vi "temperatureCheck.vi"() -> ()   [LabVIEW 2012]
uses:
  <vilib>/addons/database/Auxilliary.llb/DB Tools Cursor Type.ctl
  <vilib>/addons/database/Connection.llb/DB Tools Open Connec (Path).vi
  <vilib>/addons/database/Connection.llb/Conn Execute.vi
  <vilib>/addons/database/Recordset.llb/Rec Fetch Recordset Data (R).vi
  <vilib>/addons/database/Recordset.llb/Rec Destroy - Connection.vi
  <vilib>/addons/database/_DB Variant To Data/Database Variant To Data.xnode
  <vilib>/addons/database/NI_Database_API.lvlib
panel:
  out "error out 2":errorcluster
  out "concatenated string":string
  out "recordset data":variant[][](array[variant])
  out "error out":errorcluster
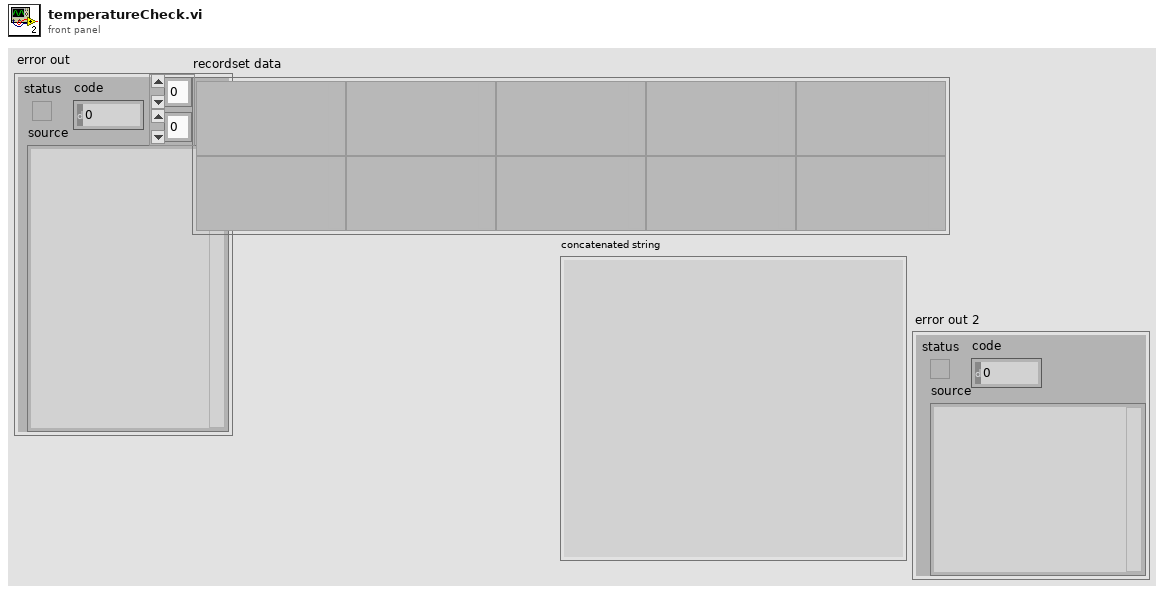
[diagram p1: front panel]
types:
  T1 = typedef "NI_Database_API.lvlib/DB Tools Cursor Type.ctl" = enum16{"forward-only", "keyset", "dynamic", "static"}
  T2 = typedef "NI_Database_API.lvlib/Conn ObjectReference.ctl" = refnum<k1>
  T3 = typedef "NI_Database_API.lvlib/Rec ObjectReference.ctl" = refnum<k1>
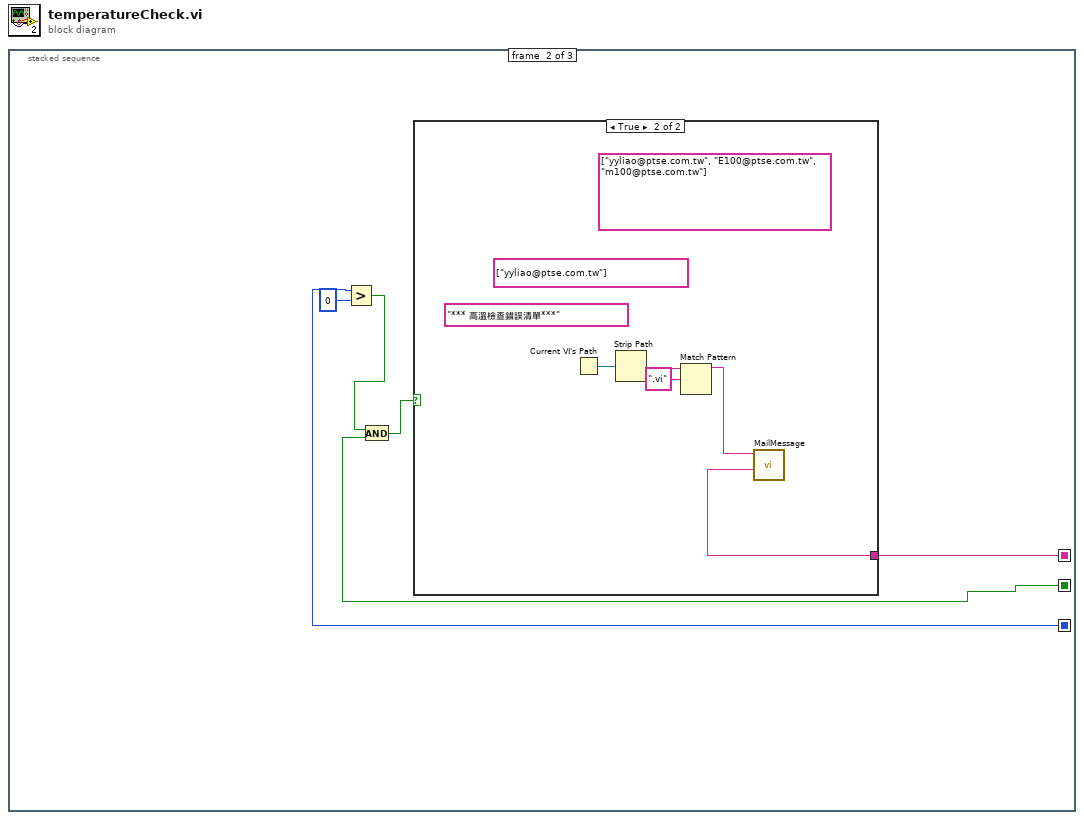
[diagram p0: block diagram]
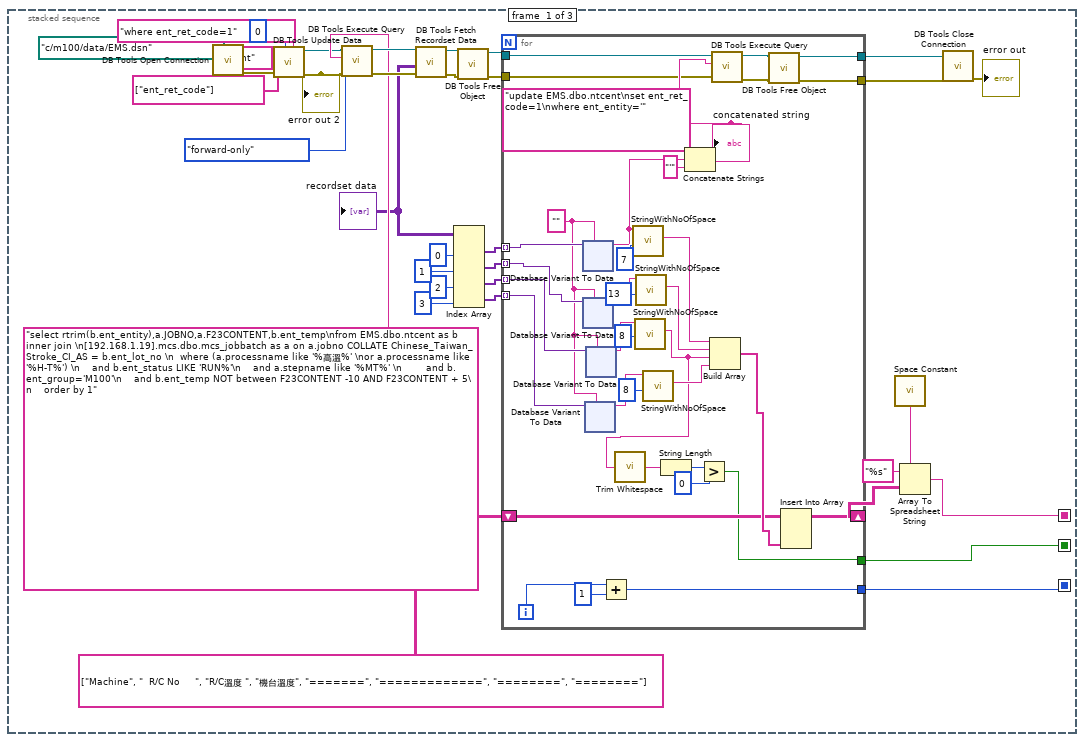
[diagram p2: hidden frame]
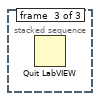
[diagram p4: hidden frame]
diagram:
  n1 = stacked-sequence {
    seq-local: [w17 _ _] -> [_ w206 _]
    seq-local: [w2 _ _] -> [_ w205 _]
    seq-local: [w1 _ _] -> [_ w201 _]
    frame #0 {
      n2 = call-poly <vilib>:"DB Tools Open Connection.vi"("connection information"=path "c:/m100/data/EMS.dsn") -> ("error out"=w8:errorcluster, "connection reference"=w10:T2)  [unwired: 7 in]
      n3 = call <vilib>:"DB Tools Update Data.vi"("condition"="where ent_ret_code=1", "data"=0, "error in (no error)"=w8, "columns"=string[] ["ent_ret_code"], "table"="ntcent", "connection reference"=w10) -> ("error out"=w7:errorcluster, "connection reference out"=w9:T2)  [unwired: 4 in]
      "error out 2" <- w7
      n4 = call-poly <vilib>:"DB Tools Execute Query.vi"("error in (no error)"=w7, "cursor type"=DB_Tools_Cursor_Type."forward-only", "SQL query"="select rtrim(b.ent_entity),a.JOBNO,a.F23CONTENT,b.ent_temp\nfrom EMS.dbo.ntcent as b inner join \n[192.168.1.19].mcs.dbo.mcs_jobbatch as a on a.jobno COLLATE Chinese_Taiwan_Stroke_CI_AS = b.ent_lot_no \n  where (a.processname like '%高溫%' \nor a.processname like '%H-T%') \n    and b.ent_status LIKE 'RUN%'\n    and a.stepname like '%MT%' \n        and b.ent_group='M100'\n    and b.ent_temp NOT between F23CONTENT -10 AND F23CONTENT + 5\n    order by 1", "connection reference"=w9) -> ("error out"=w34:errorcluster, "recordset reference"=w35:T3)  [unwired: 4 in]
      n5 = call-poly <vilib>:"DB Tools Fetch Recordset Data.vi"("error in (no error)"=w34, "recordset reference"=w35) -> ("error out"=w32:errorcluster, "recordset data"=w28:variant[][], "recordset reference out"=w33:T3)  [unwired: 3 in]
      "recordset data" <- w28
      n6 = Index Array(array=w28, index (col) #1=0 ("disabled index (col)"), index (col) #2=1 ("index (col)"), index (col) #3=2 ("index (col)"), index (col) #4=3 ("index (col)")) -> (element #1=w23:variant[], element #2=w22:variant[], element #3=w21:variant[], element #4=w20:variant[])  [unwired: 4 in]
      n7 = call-poly <vilib>:"DB Tools Free Object.vi"("error in (no error)"=w32, "recordset reference"=w33) -> ("error out"=w13:errorcluster, "connection reference"=w14:T2)  [unwired: 8 in]
      n8 = for {
        tunnel: w23 -> [w72] mode=indexing
        tunnel: w22 -> [w71] mode=indexing
        tunnel: w21 -> [w70] mode=indexing
        tunnel: w20 -> [w69] mode=indexing
        shift-right: [w66] -> w18
        shift-left: string[][] [["Machine", "  R/C No     ", "R/C溫度 ", "機台溫度"], ["=======", "=============", "========", "========"]] ("array") -> [w65]
        tunnel: w14 -> [w50]
        tunnel: w13 -> [w49]
        tunnel: [w46] -> w12
        tunnel: [w45] -> w11
        tunnel: [w42] -> w2
        tunnel: [w37] -> w1
        i -> [w44]
        w68 = ""
        n9 = xnode "Database Variant To Data"("database variant"=w72, "type"=w68) -> ("data"=w53:string)  [unwired: 1 in, 1 out]
        n10 = xnode "Database Variant To Data"("database variant"=w71, "type"=w68) -> ("data"=w57:string)  [unwired: 1 in, 1 out]
        n11 = xnode "Database Variant To Data"("database variant"=w69, "type"=w68) -> ("data"=w62:string)  [unwired: 1 in, 1 out]
        n12 = xnode "Database Variant To Data"("database variant"=w70, "type"=w68) -> ("data"=w64:string)  [unwired: 1 in, 1 out]
        n13 = Add(x=w44, y=1) -> (x+y=w42:i32)
        n14 = call "StringWithNoOfSpace.vi"("StringLength"=7, "String"=w53) -> ("OutString"=w58:string)  [unwired: 9 in]
        n15 = call "StringWithNoOfSpace.vi"("StringLength"=8, "String"=w64) -> ("OutString"=w40:string)  [unwired: 9 in]
        n16 = call <vilib>:"Trim Whitespace.vi"("string"=w40) -> ("trimmed string"=w41:string)  [unwired: 1 in]
        n17 = call "StringWithNoOfSpace.vi"("StringLength"=13, "String"=w57) -> ("OutString"=w55:string)  [unwired: 9 in]
        n18 = call "StringWithNoOfSpace.vi"("StringLength"=8, "String"=w62) -> ("OutString"=w60:string)  [unwired: 9 in]
        n19 = String Length(string=w41) -> (length=w39:i32)
        n20 = Concatenate Strings("update EMS.dbo.ntcent\nset ent_ret_code=1\nwhere ent_entity='", w53, "'" ("string")) -> (w51:string)
        "concatenated string" <- w51
        n21 = Greater?(x=w39, y=0) -> (0:w37:bool)
        n22 = Build Array(w58, w55, w40, w60) -> (w67:string[])
        n23 = call-poly <vilib>:"DB Tools Execute Query.vi"("error in (no error)"=w49, "SQL query"=w51, "connection reference"=w50) -> ("error out"=w47:errorcluster, "recordset reference"=w48:T3)  [unwired: 5 in]
        n24 = call-poly <vilib>:"DB Tools Free Object.vi"("error in (no error)"=w47, "recordset reference"=w48) -> ("error out"=w45:errorcluster, "connection reference"=w46:T2)  [unwired: 8 in]
        n25 = Insert Into Array(array=w65, new element=w67) -> (w66:string[][])  [unwired: 2 in]
      }
      n26 = call <vilib>:"Space Constant.vi"() -> ("String"=w15:string)
      n27 = Array To Spreadsheet String(delimiter (Tab)=w15, array=w18, 3:"%s" ("format string")) -> (spreadsheet string=w17:string)
      n28 = call <vilib>:"DB Tools Close Connection.vi"("error in (no error)"=w11, "connection reference"=w12) -> ("error out"=→"error out":errorcluster)  [unwired: 5 in]
    }
    frame #1 {
      n29 = Greater?(x=w205, y=0) -> (0:w203:bool)
      n30 = And(x=w203, y=w201) -> (x .and. y?=w202:bool)
      n31 = case shown="True" w202 {
        tunnel: w206 -> [_ w207]
        frame False {
        }
        frame True {
          (unwired) string[] ["yyliao@ptse.com.tw", "E100@ptse.com.tw", "m100@ptse.com.tw"] ("recipients")
          (unwired) "*** 高溫檢查錯誤清單***" ("subject ([No Subject])")
          (unwired) string[] ["yyliao@ptse.com.tw"] ("recipients")
          n32 = Current VI's Path() -> (path=w211:path)
          n33 = Strip Path(path=w211) -> (name=w210:string)  [unwired: 1 out]
          n34 = Match Pattern(string=w210, regular expression=".vi") -> (before substring=w208:string)  [unwired: 1 in, 3 out]
          n35 = call "MailMessage.vi"("message"=w207, "program"=w208) -> ()  [unwired: 10 in]
        }
      }
    }
    frame #2 {
      n36 = Quit LabVIEW() -> ()  [unwired: 1 in]
    }
  }
